vi "Configure Filter.vi"(8 "error in (no error)":errorcluster, 10 "Filter":refnum<class "Filter.lvclass">, 11 "Debug Log In":refnum<class "Debug Log.lvclass">) -> (0 "error out":errorcluster, 3 "Debug Log Out":refnum<class "Debug Log.lvclass">)   [LabVIEW 2020, in "Debug Log.lvclass"]
uses:
  Debug Log.lvclass
  Filter/Filter.lvclass
  Debug Log.lvclass/Debug Log.ctl
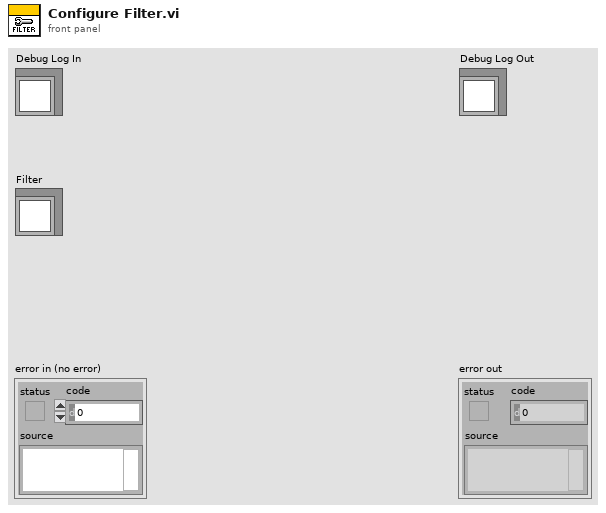
[diagram p1: front panel]
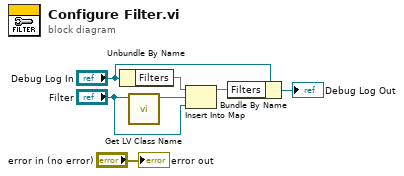
[diagram p0: block diagram]
diagram:
  n1 = Unbundle By Name("Debug Log In") -> ("Filters"=w3:map{string, refnum<class "Filter.lvclass">})
  n2 = call <vilib>:"Get LV Class Name.vi"("object"="Filter") -> ("class name"=w2:string)  [unwired: 9 in, 1 out]
  n3 = Insert Into Map(map in=w3, key=w2, value="Filter") -> (map out=w4:map{string, refnum<class "Filter.lvclass">})  [unwired: 2 out]
  n4 = Bundle By Name(cluster="Debug Log In", "Filters"=w4) -> (→"Debug Log Out":refnum<class "Debug Log.lvclass">)
  "error out" <- "error in (no error)"
